vi "1.vi"() -> ()   [LabVIEW 2016]
panel:
  out "status":bool
  out "IMAGEN ORIGINAL":picture
  out "IMAGEN MODIFICADA":picture
  out "HISTOGRAMA":dbl[][](graph)
  out "Error Out":errorcluster
  in  "IMAGEN 1":path
  in  "OPERADORES":T1 {"y 2" scale=0.0..4.0; "Meter" scale=-360.0..360.0 scale format="%#_3g"; "y" scale=-150.0..150.0; "x" scale=-150.0..150.0}
  in  "OPERACIONES":T2(ring)
  in  "Stop Button":bool
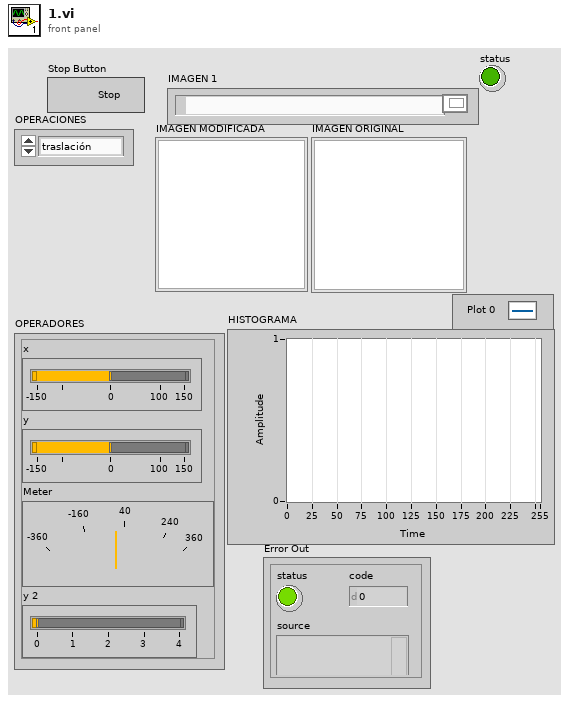
[diagram p1: front panel]
types:
  T1 = cluster{"x":dbl, "y":dbl, "Meter":dbl, "y 2":i64}
  T2 = enum16{"traslación", "Rotación", "Zoom", "GIROH", "GIROV", "Extracción", "Sustitución", "UNION"}
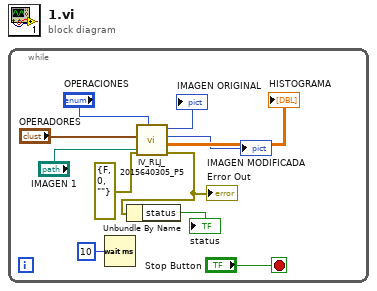
[diagram p0: block diagram]
diagram:
  n1 = while {
    stop <- "Stop Button" stop-if-true
    n2 = Wait (ms)(milliseconds to wait=u32 10) -> ()  [unwired: 1 out]
    n3 = call "IV_RLJ_2015640305_P5.vi"("OPERACIONES"="OPERACIONES", "Error In"=errorcluster {"status"=FALSE, "code"=0, "source"=""}, "OPERADORES"="OPERADORES", "IMAGEN 1"="IMAGEN 1") -> ("Error Out"=w2:errorcluster, "HISTOGRAMA"=→"HISTOGRAMA":dbl[][], "IMAGEN MODIFICADA"=→"IMAGEN MODIFICADA":picture, "IMAGEN ORIGINAL"=→"IMAGEN ORIGINAL":picture)  [unwired: 4 in]
    "Error Out" <- w2
    n4 = Unbundle By Name(w2) -> ("status"=→"status":bool)
  }
